vi "circ_ap && Zern.vi"() -> ()   [LabVIEW 2012, in "LightPipes.lvlib"]
uses:
  LightPipes.lvlib
panel:
  in  "A (Amplitude)":dbl=20.0
  in  "R( Radius)":dbl=0.0045
  in  "M (azimuthal order)":i32=2
  in  "N (radial order)":i32=2
  out "Field":cluster{"n_grid":i32, "size":dbl, "lambda":dbl}
  # "Zernlike Polynomial"
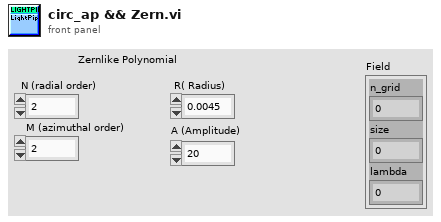
[diagram p1: front panel]
types:
  T1 = cluster{"n_grid":i32, "@dummy control@":i8, "@dummy control@":i8, "@dummy control@":i8, "@dummy control@":i8, "size":dbl, "lambda":dbl, "int1":i32, "int2":i32, "int3":i32, "@dummy control@":i8, "@dummy control@":i8, "@dummy control@":i8, "@dummy control@":i8, "double1":dbl, "double2":dbl, "double3":dbl, "real":u32, "imaginary":u32}
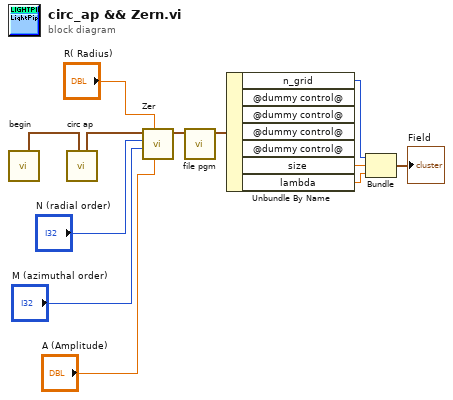
[diagram p0: block diagram]
diagram:
  n1 = call "begin.vi"() -> ("field out"=w9:T1)  [unwired: 11 in]
  n2 = call "circ ap.vi"("field"=w9) -> ("field out"=w8:T1)  [unwired: 10 in]
  n3 = call "Zer.vi"("A (Amplitude)"="A (Amplitude)", "R( Radius)"="R( Radius)", "M (azimuthal order)"="M (azimuthal order)", "N (radial order)"="N (radial order)", "field"=w8) -> ("field out"=w3:T1)  [unwired: 6 in]
  n4 = call "file pgm.vi"("field"=w3) -> ("field out"=w2:T1)  [unwired: 9 in, 1 out]
  n5 = Unbundle By Name(w2) -> ("n_grid"=w10:i32, "size"=w11:dbl, "lambda"=w12:dbl)  [unwired: 4 out]
  n6 = Bundle("n_grid"=w10, "size"=w11, "lambda"=w12) -> (→"Field":cluster{"n_grid":i32, "size":dbl, "lambda":dbl})  [unwired: 1 in]
